vi "Generate Waveforms.vi"(1 "Recorded Sound.lvclass":refnum<class "Recorded Sound.lvclass">=refnum) -> (0 "Waveforms":waveform(dbl)[](array[waveform]))   [LabVIEW 2010, in "Recorded Sound.lvclass"]
uses:
  Recorded Sound.lvclass
  Recorded Sound.lvclass/Recorded Sound.ctl
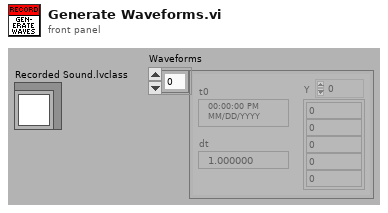
[diagram p1: front panel]
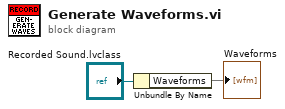
[diagram p0: block diagram]
diagram:
  n1 = Unbundle By Name("Recorded Sound.lvclass") -> ("Waveforms"=→"Waveforms")
